vi "update data reducer and NS write trigger.vi"(10 "Data 3":T1, 11 "Data in":variant) -> (2 "Data out":T1)   [LabVIEW 2018]
uses:
  <vilib>/rvi/interface/nirviReadWriteControl/nirviReadWriteControl.xnode
  Type Defs/FPGA reference.ctl
  <vilib>/rvi/interface/Simulation/niFpgaSimulationCallBeginRW.vi
  <vilib>/rvi/errors/niLvFpgaAdjustHostInterfaceError.vi
  Type Defs/Data processing loop data.ctl
  Type Defs/channelScalingTypes.ctl
  Type Defs/scalingMethods.ctl
  Type Defs/channelCalibration.ctl
panel:
  out "write trigger":u16
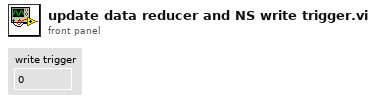
[diagram p1: front panel]
types:
  T1 = typedef "Data processing loop data.ctl" = cluster{"Parameters":cluster{"FPGA Ref":T2, "data stream":cluster{"data writer name":string, "NS write buffer size":i32, "NS Buffer length":u32}, "FIFO Depth":u32, "Channel controls":cluster{"FIFIO channel count":i32, "active indices":i16[], "active channels":i32, "channelScaling":T3[], "scanivalveCount":i32}, "safetyChannels":cluster{"oilP":u16, "airP":u16, "water":u16, "temperatures":cluster{"Oil pressure: 4":u16, "Enabled":bool, "warning temp":dbl, "limit temp":dbl, "Invert":bool}[]}}, "Variables":cluster{"Intermediary buffer":dbl[][], "buffer position":u32, "write loop counter":u16, "NS write trigger":u32, "NS Connection status":bool, "waiting for NS":bool, "labAmbient":cluster{"pressure":dbl, "temperature":dbl}, "scanivalvePorts":u16[], "scanivalvePressures":dbl[], "data stream":refnum<k21>}}
  T2 = typedef "FPGA reference.ctl" = refnum<k20>
  T3 = typedef "channelCalibration.ctl" = cluster{"index":u16, "active":bool, "channelType":T4, "module":u16, "terminal":u16, "channelName":string, "scalingMethod":T5, "scalingParameters":dbl[], "scaledUnits":string}
  T4 = typedef "channelScalingTypes.ctl" = enum16{"calculation", "measurement", "scanivalve", "output", "digital"}
  T5 = typedef "scalingMethods.ctl" = enum16{"none", "linear", "thermocouple", "polynomial", "encoder", "RTD"}
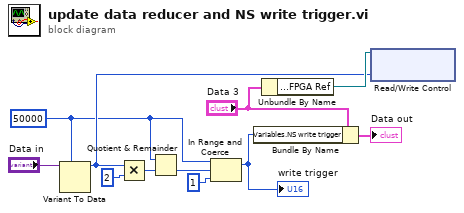
[diagram p0: block diagram]
diagram:
  w4 = u16 50000 ("data reducer")
  n1 = Variant To Data(type=w4, Variant="Data in") -> (data=w7:u16)  [unwired: 1 in, 1 out]
  n2 = Multiply(x=w7, y=u16 2) -> (x*y=w2:u16)
  n3 = Quotient & Remainder(x=w4, y=w2) -> (floor(x/y)=w6:u16)  [unwired: 1 out]
  n4 = In Range and Coerce(upper limit=w4, x=w6, lower limit=u16 1) -> (coerced(x)=w3:u16)  [unwired: 1 out]
  "write trigger" <- w3
  n5 = Bundle By Name(cluster="Data 3", "Variables.NS write trigger"=w3) -> (→"Data out":T1)
  n6 = Unbundle By Name("Data 3") -> ("Parameters.FPGA Ref"=w9:T2)
  n7 = xnode "Read/Write Control"("FPGA VI Reference In"=w9, "data reducer"=w7) -> ()  [unwired: 1 in, 2 out]
